vi "m10.wf.compose.test.vi"() -> ()   [LabVIEW 2012]
panel:
  in  "Waveform Properties":T1={"Fs (Hz)"=20000.0, "Amplitude (V)"=5.0, "Ramp (s)"=0.02} {"Ramp (s)" min=0.0; "Fs (Hz)" min=0.0}
  in  "Repetitions":T2={"Rep type"=1, "Duration (s)"=0.25, "Delay (s)"=0.0, "Interval (s)"=0.0, "M"=1} {"Rep type" items=["Off", "DC", "Trig", "Train", "Gate"]}
  out "Digital Waveform":digitalwaveform(graph)={"t0"=timestamp(0 s since 1904-01-01), "dt"=5e-05, "Y"={"transitions"=[], "data"=array5000x1[5000 elements]}}
  in  "WF Dur (s)":dbl=0.5
  out "Analog Waveform":waveform(dbl)(graph)={"t0"=timestamp(0 s since 1904-01-01), "dt"=5e-05, "Y"=array[9999 elements]}
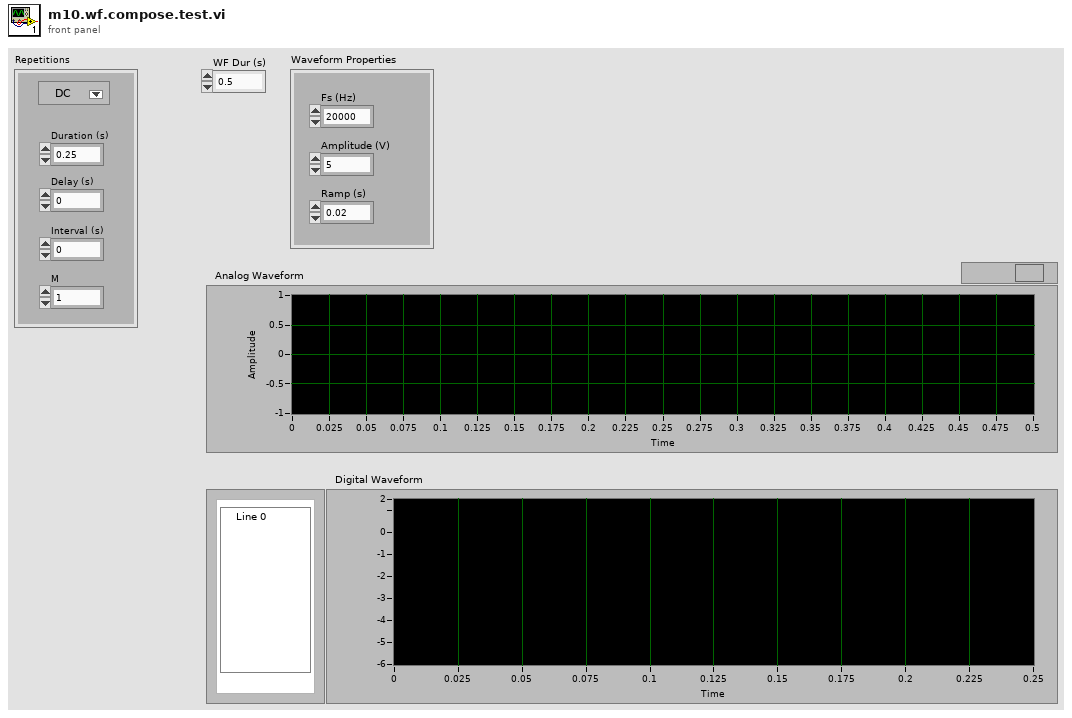
[diagram p1: front panel]
types:
  T1 = cluster{"Fs (Hz)":dbl, "Amplitude (V)":dbl, "Ramp (s)":dbl}
  T2 = cluster{"Rep type":u16, "Duration (s)":dbl, "Delay (s)":dbl, "Interval (s)":dbl, "M":i32}
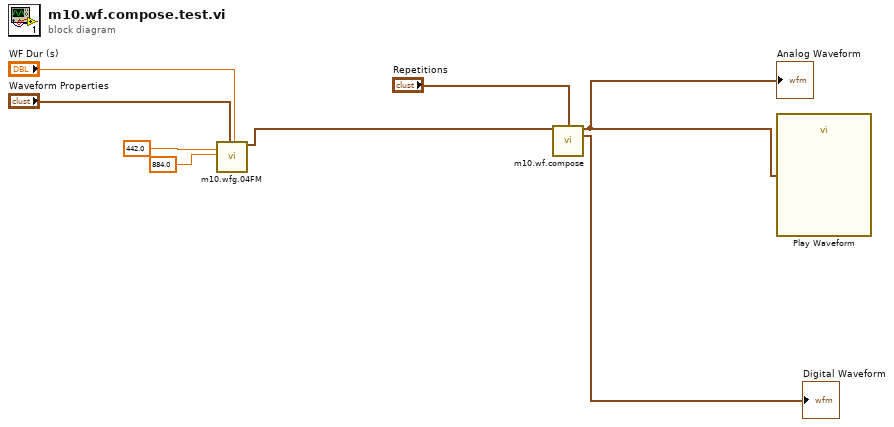
[diagram p0: block diagram]
diagram:
  n1 = call "m10.wfg.04FM.vi"("Param 0"=442.0, "Param 1"=884.0, "Waveform Properties"="Waveform Properties", "Duration (s)"="WF Dur (s)") -> ("Waveform Out"=w1:waveform(dbl))  [unwired: 14 in, 1 out]
  n2 = call "m10.wf.compose.vi"("Waveform In"=w1, "Repetitions"="Repetitions") -> ("Analog Waveform Out"=w8:waveform(dbl), "Digital Waveform Out"=→"Digital Waveform":digitalwaveform)  [unwired: 11 in, 1 out]
  "Analog Waveform" <- w8
  n3 = call "Play Waveform"("Data"=w8) -> ()  [unwired: 18 in, 1 out]
